vi "Get Self.vi"(11 "Queue Mailbox in":refnum<class "Queue Mailbox.lvclass">) -> (2 "Self":refnum<data-value>)   [LabVIEW 2021, in "jettl.lvlib" / "Mailbox.lvlib" / "Queue Mailbox.lvclass"]
uses:
  Queue Mailbox.lvclass
  Msg Strategy/Msg Strategy.lvclass
  Queue Mailbox.lvclass/Queue Mailbox.ctl
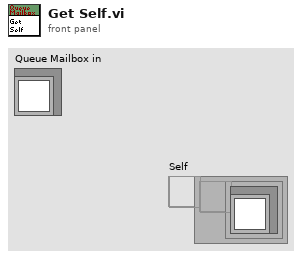
[diagram p1: front panel]
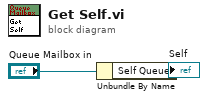
[diagram p0: block diagram]
diagram:
  n1 = Unbundle By Name("Queue Mailbox in") -> ("Self Queue"=→"Self":refnum<data-value>)
